vi "XOR Plain Text with Non-Random Key.vi"() -> ()   [LabVIEW 2016]
panel:
  out "Plaintext Distribution":dynamicdata(graph) caption="Histogram"
  out "Cipher Distribution":dynamicdata(graph) caption="Histogram"
  out "Key Distyribution":dynamicdata(graph) caption="Histogram"
  out "Deciphered Text":string="Hello LabVIEW World!"
  in  "Key":string="Jim's secret (Shhh!)"
  out "Cipher Text":string
  in  "Plain Text":string="Hello LabVIEW World!"
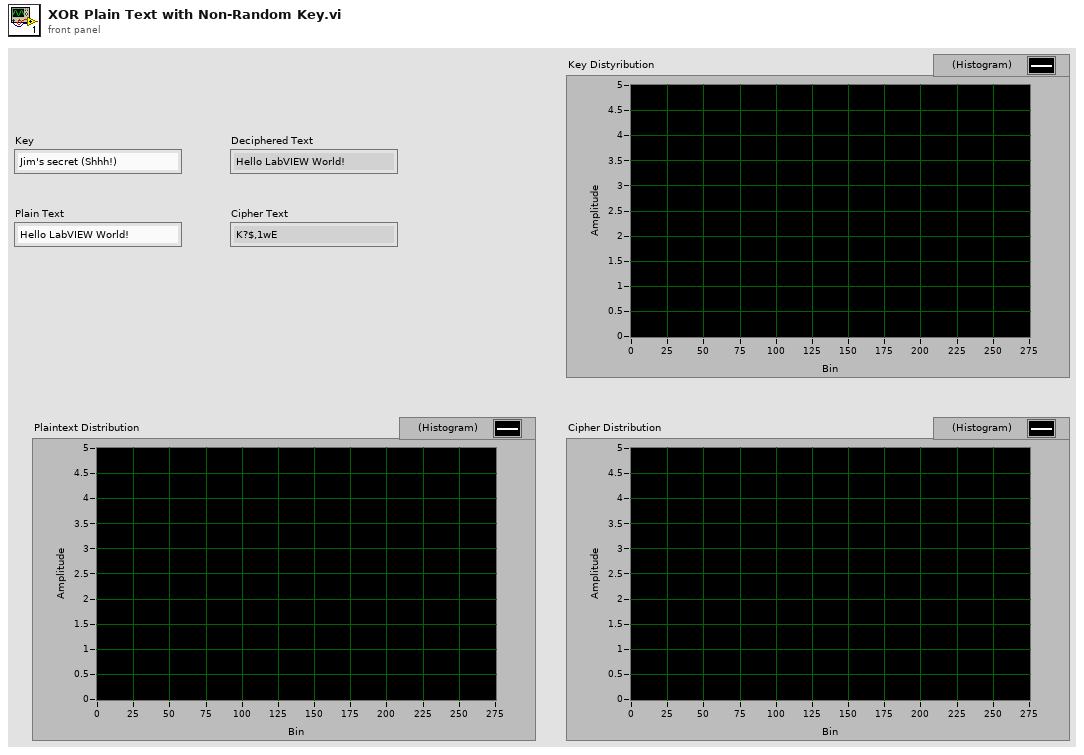
[diagram p1: front panel]
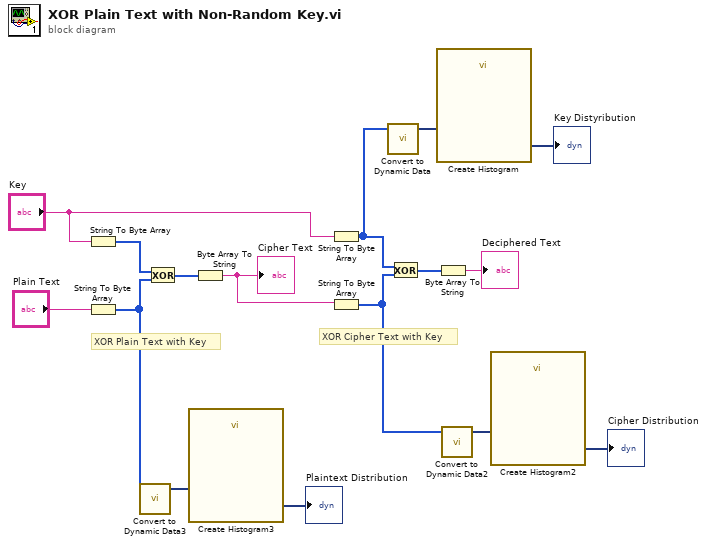
[diagram p0: block diagram]
diagram:
  # "XOR Cipher Text with Key"
  # "XOR Plain Text with Key"
  n1 = String To Byte Array(string="Key") -> (unsigned byte array=w16:u8[])
  n2 = String To Byte Array(string="Plain Text") -> (unsigned byte array=w1:u8[])
  n3 = call "Convert to Dynamic Data3"("Array"=w1) -> ("Dynamic Data Type"=w3:dynamicdata)  [unwired: 3 in]
  n4 = Exclusive Or(1:w1, 2:w16) -> (0:w14:u8[])
  n5 = call "Create Histogram3"("Signal"=w3) -> ("Histogram"=→"Plaintext Distribution":dynamicdata)  [unwired: 9 in, 1 out]
  n6 = Byte Array To String(unsigned byte array=w14) -> (string=w13:string)
  "Cipher Text" <- w13
  n7 = String To Byte Array(string="Key") -> (unsigned byte array=w8:u8[])
  n8 = String To Byte Array(string=w13) -> (unsigned byte array=w4:u8[])
  n9 = call "Convert to Dynamic Data"("Array"=w8) -> ("Dynamic Data Type"=w10:dynamicdata)  [unwired: 3 in]
  n10 = Exclusive Or(1:w4, 2:w8) -> (0:w5:u8[])
  n11 = call "Create Histogram"("Signal"=w10) -> ("Histogram"=→"Key Distyribution":dynamicdata)  [unwired: 9 in, 1 out]
  n12 = Byte Array To String(unsigned byte array=w5) -> (string=→"Deciphered Text":string)
  n13 = call "Convert to Dynamic Data2"("Array"=w4) -> ("Dynamic Data Type"=w6:dynamicdata)  [unwired: 3 in]
  n14 = call "Create Histogram2"("Signal"=w6) -> ("Histogram"=→"Cipher Distribution":dynamicdata)  [unwired: 9 in, 1 out]
